vi "bumper d.vi"() -> ()   [LabVIEW 2013]
uses:
  <vilib>/NXT/Block Support/NXT_InputPort.ctl
  <vilib>/NXT/Block Support/NXT_MessageMailbox.ctl
  <vilib>/NXT/Subs/MotorOutput.ctl
  <vilib>/NXT/Block Support/NXT_OutputPort.ctl
  <vilib>/NXT/Dual Mode Library/BT/BlueTooth_Write_Num.vi
  <vilib>/NXT/Dual Mode Library/Display/drawNumber_float.vi
  <vilib>/NXT/Dual Mode Library/Display/drawNumber.vi
  <vilib>/NXT/Dual Mode Library/Sound/PlayRedPianoFile.vi
  <vilib>/NXT/NXTIO Xnodes/NXTIONodeSubVIs/NXTStopMotors.vi
  <vilib>/NXT/NXTIO Xnodes/AddressXNode/NXTIOAddress.xnode
  <vilib>/NXT/NXTIO Xnodes/NXTIOXNode/NXTIO.xnode
  <vilib>/NXT/Subs/LVHSConnector.ctl
  <vilib>/NXT/LegoClasses/BrickReference/BrickReference.lvclass
panel:
  out "Case Accord. BJr.":i32
  out "touch right":bool
  out "touch left":bool
  in  "threshold steer":dbl=0.2
  out "norm dist":dbl
  out "right dist":i16
  out "left dist":i16
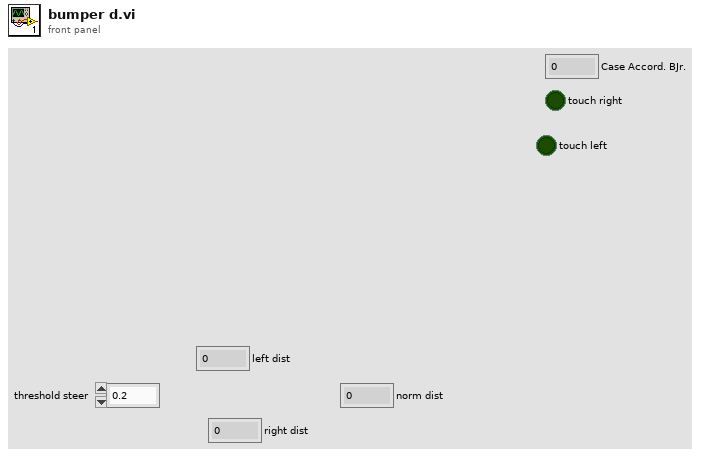
[diagram p1: front panel]
types:
  T1 = typedef "NXT_OutputPort.ctl" = u8
  T2 = typedef "NXT_MessageMailbox.ctl" = u8
  T3 = typedef "NXT_InputPort.ctl" = u32
  T4 = typedef "LVHSConnector.ctl" = refnum<class "BrickReference.lvclass">
  T5 = typedef "MotorOutput.ctl" = u8
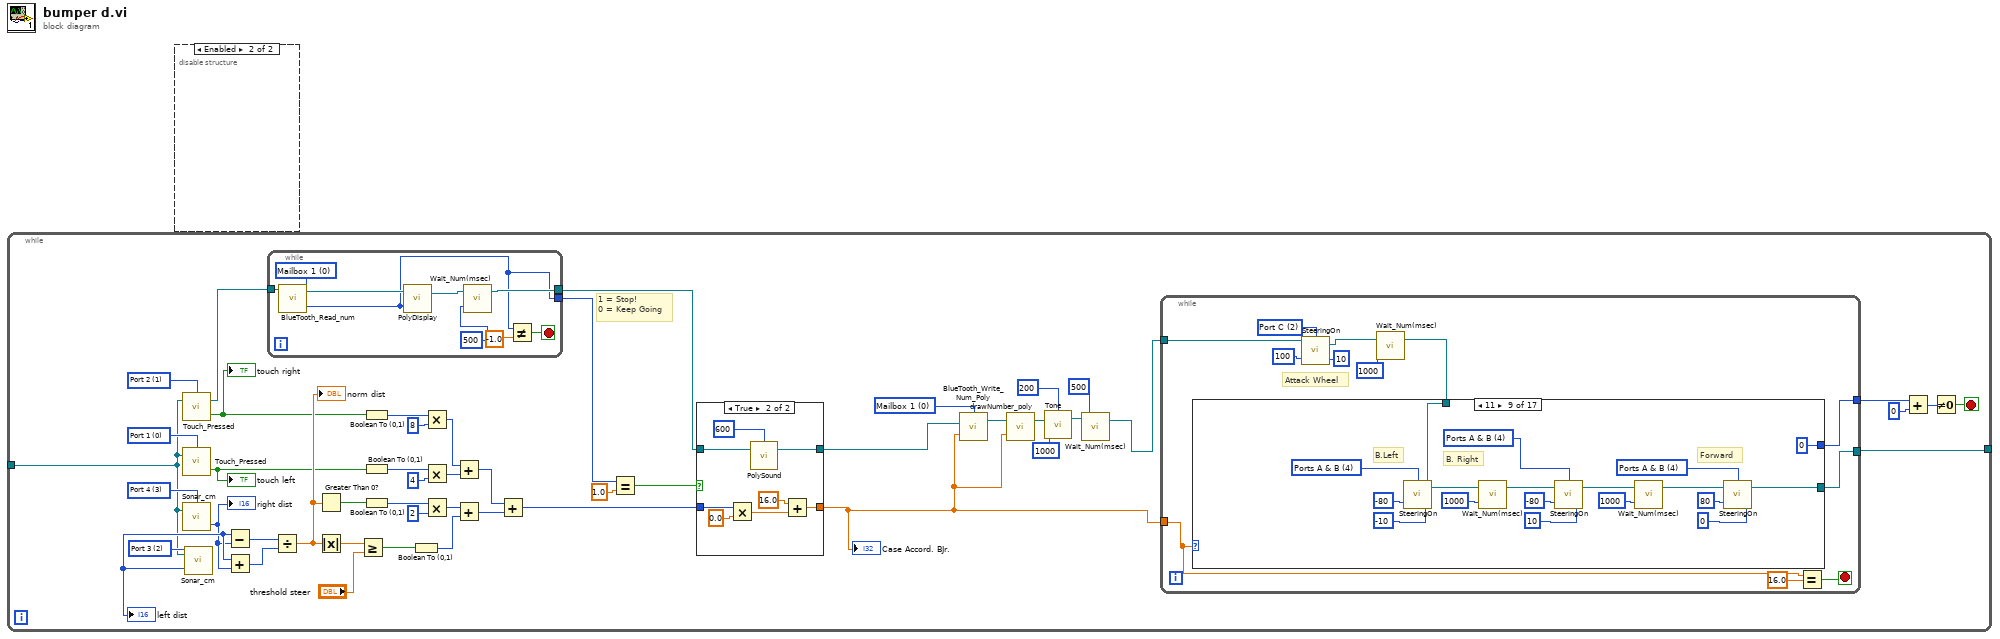
[diagram p0: block diagram]
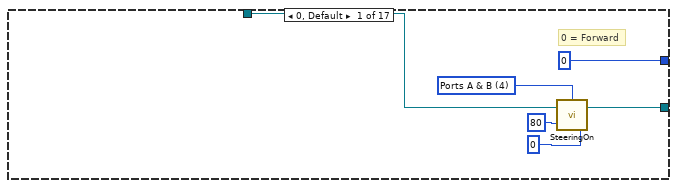
[diagram p3: hidden frame]
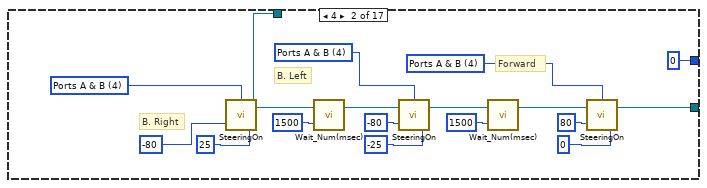
[diagram p4: hidden frame]
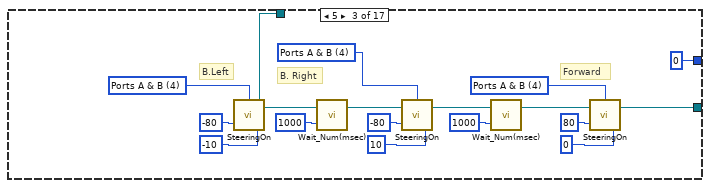
[diagram p5: hidden frame]
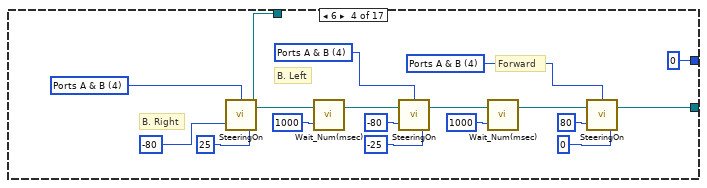
[diagram p6: hidden frame]
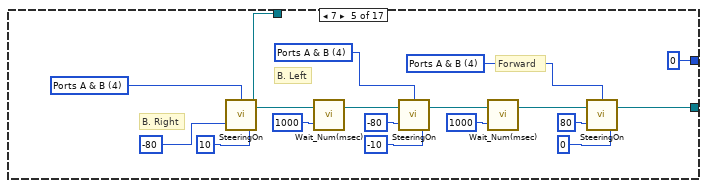
[diagram p7: hidden frame]
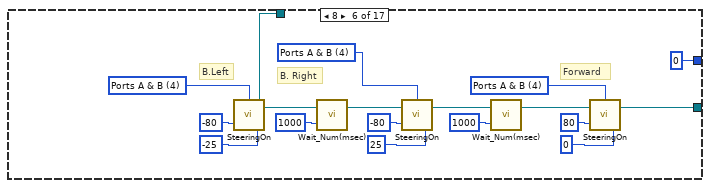
[diagram p8: hidden frame]
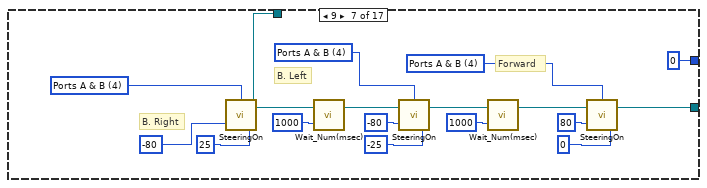
[diagram p9: hidden frame]
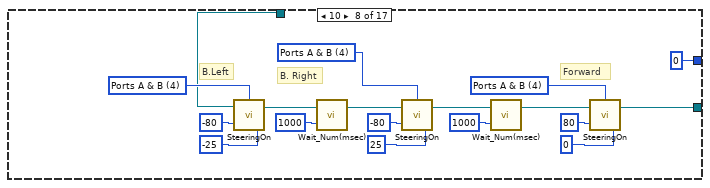
[diagram p10: hidden frame]
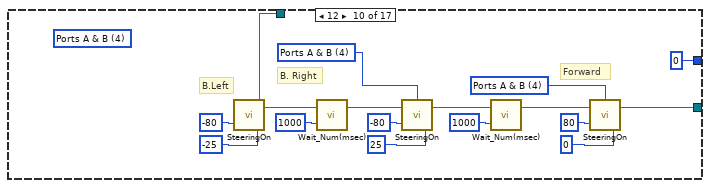
[diagram p11: hidden frame]
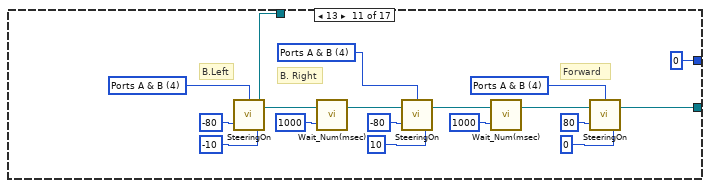
[diagram p12: hidden frame]
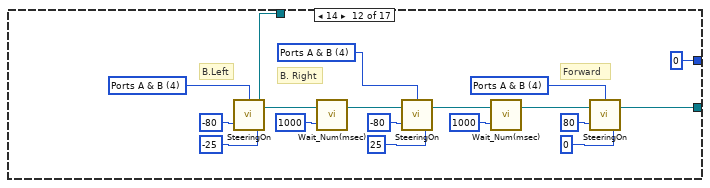
[diagram p13: hidden frame]
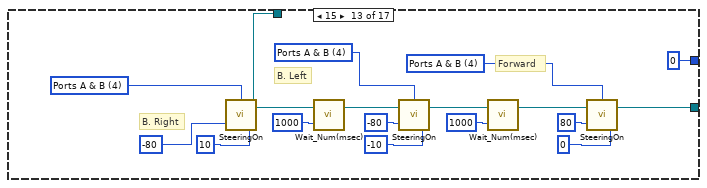
[diagram p14: hidden frame]
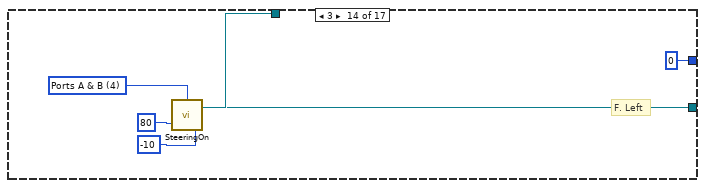
[diagram p15: hidden frame]
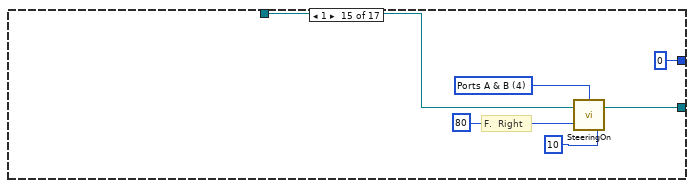
[diagram p16: hidden frame]
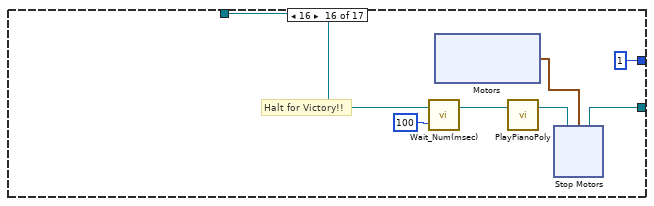
[diagram p17: hidden frame]
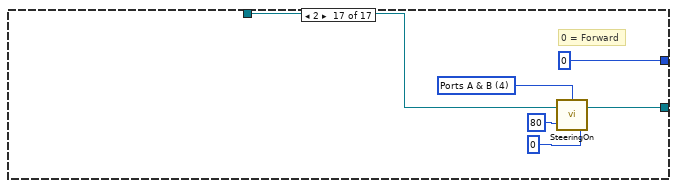
[diagram p18: hidden frame]
diagram:
  n1 = while {
    tunnel: [w15] -> _
    tunnel: [w5] -> _
    stop <- w17 stop-if-true
    w11 = T2 0 items=["Mailbox 1", "Mailbox 2", "Mailbox 3", "Mailbox 4", "Mailbox 5", "Mailbox 6", "Mailbox 7", "Mailbox 8", "Mailbox 9", "Mailbox 10"] ("Mailbox")
    w39 = T3 1 items=["Port 1", "Port 2", "Port 3", "Port 4"] ("Port (Port 1)")
    w40 = T3 0 items=["Port 1", "Port 2", "Port 3", "Port 4"] ("Port (Port 1)")
    w48 = T3 3 items=["Port 1", "Port 2", "Port 3", "Port 4"] ("Port (Port 4)")
    w49 = T3 2 items=["Port 1", "Port 2", "Port 3", "Port 4"] ("Port (Port 4)")
    # "1 = Stop!\n0 = Keep Going"
    n2 = call <vilib>:"Sonar_cm.vi"("Port (Port 4)"=w49) -> ("Distance (cm)"=w47:i16, "NXT/EV3"=w15:T4)  [unwired: 2 in]
    "left dist" <- w47
    n3 = call <vilib>:"Touch_Pressed.vi"("NXT/EV3"=w15, "Port (Port 1)"=w39) -> ("Yes / No"=w25:bool, "NXT/EV3"=w13:T4)  [unwired: 1 in]
    "touch right" <- w25
    n4 = call <vilib>:"Touch_Pressed.vi"("NXT/EV3"=w15, "Port (Port 1)"=w40) -> ("Yes / No"=w26:bool)  [unwired: 1 in, 1 out]
    "touch left" <- w26
    n5 = call <vilib>:"Sonar_cm.vi"("NXT/EV3"=w15, "Port (Port 4)"=w48) -> ("Distance (cm)"=w46:i16)  [unwired: 1 in, 1 out]
    "right dist" <- w46
    n6 = Subtract(x=w47, y=w46) -> (x-y=w45:i16)
    n7 = Add(x=w47, y=w46) -> (x+y=w44:i16)
    n8 = while {
      tunnel: w13 -> [w318]
      tunnel: [w314] -> w21
      tunnel: [w315] -> w14
      stop <- w321 stop-if-true
      w317 = T2 0 items=["Mailbox 1", "Mailbox 2", "Mailbox 3", "Mailbox 4", "Mailbox 5", "Mailbox 6", "Mailbox 7", "Mailbox 8", "Mailbox 9", "Mailbox 10"] ("Mailbox")
      n9 = call <vilib>:"BlueTooth_Read_num.vi"("NXT/EV3"=w318, "Mailbox"=w317) -> ("Message"=w314:i32, "NXT/EV3"=w320:T4)  [unwired: 1 in]
      n10 = call-poly <vilib>:"PolyDisplay.vi"("number"=w314, "NXT/EV3"=w320) -> ("NXT/EV3"=w319:T4)  [unwired: 2 in]
      n11 = call <vilib>:"Wait_Num(msec).vi"("Time (100 msec)"=u32 500, "NXT/EV3"=w319) -> ("NXT/EV3"=w315:T4)  [unwired: 2 in]
      n12 = Not Equal?(x=w314, y=-1.0) -> (x != y?=w321:bool)
    }
    n13 = Divide(x=w45, y=w44) -> (x/y=w41:dbl)
    "norm dist" <- w41
    n14 = Greater Than 0?(x=w41) -> (x > 0?=w24:bool)
    n15 = Absolute Value(x=w41) -> (abs(x)=w43:dbl)
    n16 = Greater Or Equal?(x=w43, y="threshold steer") -> (x >= y?=w23:bool)
    n17 = Boolean To (0,1)(Boolean=w25) -> (0, 1=w34:i16)
    n18 = Boolean To (0,1)(Boolean=w26) -> (0, 1=w33:i16)
    n19 = Boolean To (0,1)(Boolean=w24) -> (0, 1=w38:i16)
    n20 = Boolean To (0,1)(Boolean=w23) -> (0, 1=w28:i16)
    n21 = Multiply(x=w34, y=i16 8) -> (x*y=w31:i16)
    n22 = Multiply(x=w33, y=i16 4) -> (x*y=w30:i16)
    n23 = Multiply(x=w38, y=i16 2) -> (x*y=w29:i16)
    n24 = Add(x=w31, y=w30) -> (x+y=w32:i16)
    n25 = Add(x=w29, y=w28) -> (x+y=w27:i16)
    n26 = Add(x=w32, y=w27) -> (x+y=w16:i16)
    n27 = Equal?(x=w21, y=1.0) -> (x = y?=w20:bool)
    n28 = case shown="True" w20 {
      tunnel: w16 -> [w324 w330]
      tunnel: [w324 w325] -> w7
      tunnel: w14 -> [w323 w329]
      tunnel: [w323 w328] -> w9
      frame False {
      }
      frame True {
        n29 = Multiply(x=w330, y=0.0) -> (x*y=w327:dbl)
        n30 = call-poly <vilib>:"PolySound.vi"("NXT/EV3"=w329, "Tone (440 Hz)"=u16 600) -> ("NXT/EV3"=w328:T4)  [unwired: 2 in]
        n31 = Add(x=16.0, y=w327) -> (x+y=w325:dbl)
      }
    }
    "Case Accord. BJr." <- w7
    n32 = call-poly <vilib>:"BlueTooth_Write_Num_Poly.vi"("Message"=w7, "NXT/EV3"=w9, "Mailbox"=w11) -> ("NXT/EV3"=w12:T4)  [unwired: 1 in]
    n33 = call-poly <vilib>:"drawNumber_poly.vi"("number"=w7, "NXT/EV3"=w12) -> ("NXT/EV3"=w3:T4)  [unwired: 2 in]
    n34 = call <vilib>:"Tone.vi"("Duration (500 ms)"=u16 1000, "NXT/EV3"=w3, "Tone (440 Hz)"=u16 200) -> ("NXT/EV3"=w2:T4)  [unwired: 1 in]
    n35 = call <vilib>:"Wait_Num(msec).vi"("Time (100 msec)"=u32 500, "NXT/EV3"=w2) -> ("NXT/EV3"=w8:T4)  [unwired: 2 in]
    n36 = while {
      tunnel: w8 -> [w58]
      tunnel: w7 -> [w53]
      tunnel: [w57] -> w6
      tunnel: [w56] -> w5
      stop <- w55 stop-if-true
      w61 = T5 2 items=["Port A"=0, "Port B"=1, "Port C"=2, "Ports A & B"=4, "Ports A & C"=5, "Ports B & C"=6, "All Ports"=3] ("Output Ports (A & B)")
      # "Attack Wheel"
      n37 = call <vilib>:"SteeringOn.vi"("Power (75)"=100, "Steering (100)"=10, "NXT/EV3"=w58, "Output Ports (A & B)"=w61) -> ("NXT/EV3"=w52:T4)
      n38 = call <vilib>:"Wait_Num(msec).vi"("Time (100 msec)"=u32 1000, "NXT/EV3"=w52) -> ("NXT/EV3"=w51:T4)  [unwired: 2 in]
      n39 = case shown="11" w53 {
        tunnel: w51 -> [w65 w79 w88 w106 w124 w151 w160 w178 w196 w214 w231 w249 w268 w286 w292 w295 w311]
        tunnel: [w64 w78 w87 w105 w123 w150 w159 w177 w195 w213 w230 w248 w267 w285 w291 w298 w310] -> w56
        tunnel: [0 ("y") 0 ("y") 0 ("y") 0 ("y") 0 ("y") 0 ("y") 0 ("y") 0 ("y") 0 ("y") 0 ("y") 0 ("y") 0 ("y") 0 ("y") 0 ("y") 0 1 0 ("y")] -> w57
        frame 0, Default {
          w63 = T5 4 items=["Port A"=0, "Port B"=1, "Port C"=2, "Ports A & B"=4, "Ports A & C"=5, "Ports B & C"=6, "All Ports"=3] ("Output Ports (A & B) 5")
          # "0 = Forward"
          n40 = call <vilib>:"SteeringOn.vi"("Power (75)"=80, "Steering (100)"=0, "NXT/EV3"=w65, "Output Ports (A & B)"=w63) -> ("NXT/EV3"=w64:T4)
        }
        frame 4 {
          w75 = T5 4 items=["Port A"=0, "Port B"=1, "Port C"=2, "Ports A & B"=4, "Ports A & C"=5, "Ports B & C"=6, "All Ports"=3] ("Output Ports (A & B) 15")
          w76 = T5 4 items=["Port A"=0, "Port B"=1, "Port C"=2, "Ports A & B"=4, "Ports A & C"=5, "Ports B & C"=6, "All Ports"=3] ("Output Port (All Ports) 6")
          w77 = T5 4 items=["Port A"=0, "Port B"=1, "Port C"=2, "Ports A & B"=4, "Ports A & C"=5, "Ports B & C"=6, "All Ports"=3] ("Output Ports (A & B) 16")
          # "Forward"
          # "B. Left"
          # "B. Right"
          n41 = call <vilib>:"SteeringOn.vi"("Power (75)"=-80, "Steering (100)"=25, "NXT/EV3"=w79, "Output Ports (A & B)"=w77) -> ("NXT/EV3"=w74:T4)
          n42 = call <vilib>:"Wait_Num(msec).vi"("Time (100 msec)"=u32 1500, "NXT/EV3"=w74) -> ("NXT/EV3"=w73:T4)  [unwired: 2 in]
          n43 = call <vilib>:"SteeringOn.vi"("Power (75)"=-80, "Steering (100)"=-25, "NXT/EV3"=w73, "Output Ports (A & B)"=w76) -> ("NXT/EV3"=w72:T4)
          n44 = call <vilib>:"Wait_Num(msec).vi"("Time (100 msec)"=u32 1500, "NXT/EV3"=w72) -> ("NXT/EV3"=w71:T4)  [unwired: 2 in]
          n45 = call <vilib>:"SteeringOn.vi"("Power (75)"=80, "Steering (100)"=0, "NXT/EV3"=w71, "Output Ports (A & B)"=w75) -> ("NXT/EV3"=w78:T4)
        }
        frame 5 {
          w95 = T5 4 items=["Port A"=0, "Port B"=1, "Port C"=2, "Ports A & B"=4, "Ports A & C"=5, "Ports B & C"=6, "All Ports"=3] ("Output Ports (A & B) 21")
          w96 = T5 4 items=["Port A"=0, "Port B"=1, "Port C"=2, "Ports A & B"=4, "Ports A & C"=5, "Ports B & C"=6, "All Ports"=3] ("Output Port (All Ports) 9")
          w97 = T5 4 items=["Port A"=0, "Port B"=1, "Port C"=2, "Ports A & B"=4, "Ports A & C"=5, "Ports B & C"=6, "All Ports"=3] ("Output Ports (A & B) 22")
          # "Forward"
          # "B. Right"
          # "B.Left"
          n46 = call <vilib>:"SteeringOn.vi"("Power (75)"=-80, "Steering (100)"=-10, "NXT/EV3"=w88, "Output Ports (A & B)"=w97) -> ("NXT/EV3"=w93:T4)
          n47 = call <vilib>:"Wait_Num(msec).vi"("Time (100 msec)"=u32 1000, "NXT/EV3"=w93) -> ("NXT/EV3"=w92:T4)  [unwired: 2 in]
          n48 = call <vilib>:"SteeringOn.vi"("Power (75)"=-80, "Steering (100)"=10, "NXT/EV3"=w92, "Output Ports (A & B)"=w96) -> ("NXT/EV3"=w90:T4)
          n49 = call <vilib>:"Wait_Num(msec).vi"("Time (100 msec)"=u32 1000, "NXT/EV3"=w90) -> ("NXT/EV3"=w89:T4)  [unwired: 2 in]
          n50 = call <vilib>:"SteeringOn.vi"("Power (75)"=80, "Steering (100)"=0, "NXT/EV3"=w89, "Output Ports (A & B)"=w95) -> ("NXT/EV3"=w87:T4)
        }
        frame 6 {
          w115 = T5 4 items=["Port A"=0, "Port B"=1, "Port C"=2, "Ports A & B"=4, "Ports A & C"=5, "Ports B & C"=6, "All Ports"=3] ("Output Ports (A & B) 15")
          w114 = T5 4 items=["Port A"=0, "Port B"=1, "Port C"=2, "Ports A & B"=4, "Ports A & C"=5, "Ports B & C"=6, "All Ports"=3] ("Output Port (All Ports) 6")
          w113 = T5 4 items=["Port A"=0, "Port B"=1, "Port C"=2, "Ports A & B"=4, "Ports A & C"=5, "Ports B & C"=6, "All Ports"=3] ("Output Ports (A & B) 16")
          # "Forward"
          # "B. Left"
          # "B. Right"
          n51 = call <vilib>:"SteeringOn.vi"("Power (75)"=-80, "Steering (100)"=25, "NXT/EV3"=w106, "Output Ports (A & B)"=w113) -> ("NXT/EV3"=w116:T4)
          n52 = call <vilib>:"Wait_Num(msec).vi"("Time (100 msec)"=u32 1000, "NXT/EV3"=w116) -> ("NXT/EV3"=w117:T4)  [unwired: 2 in]
          n53 = call <vilib>:"SteeringOn.vi"("Power (75)"=-80, "Steering (100)"=-25, "NXT/EV3"=w117, "Output Ports (A & B)"=w114) -> ("NXT/EV3"=w118:T4)
          n54 = call <vilib>:"Wait_Num(msec).vi"("Time (100 msec)"=u32 1000, "NXT/EV3"=w118) -> ("NXT/EV3"=w119:T4)  [unwired: 2 in]
          n55 = call <vilib>:"SteeringOn.vi"("Power (75)"=80, "Steering (100)"=0, "NXT/EV3"=w119, "Output Ports (A & B)"=w115) -> ("NXT/EV3"=w105:T4)
        }
        frame 7 {
          w133 = T5 4 items=["Port A"=0, "Port B"=1, "Port C"=2, "Ports A & B"=4, "Ports A & C"=5, "Ports B & C"=6, "All Ports"=3] ("Output Ports (A & B) 15")
          w132 = T5 4 items=["Port A"=0, "Port B"=1, "Port C"=2, "Ports A & B"=4, "Ports A & C"=5, "Ports B & C"=6, "All Ports"=3] ("Output Port (All Ports) 6")
          w131 = T5 4 items=["Port A"=0, "Port B"=1, "Port C"=2, "Ports A & B"=4, "Ports A & C"=5, "Ports B & C"=6, "All Ports"=3] ("Output Ports (A & B) 16")
          # "Forward"
          # "B. Left"
          # "B. Right"
          n56 = call <vilib>:"SteeringOn.vi"("Power (75)"=-80, "Steering (100)"=10, "NXT/EV3"=w124, "Output Ports (A & B)"=w131) -> ("NXT/EV3"=w134:T4)
          n57 = call <vilib>:"Wait_Num(msec).vi"("Time (100 msec)"=u32 1000, "NXT/EV3"=w134) -> ("NXT/EV3"=w135:T4)  [unwired: 2 in]
          n58 = call <vilib>:"SteeringOn.vi"("Power (75)"=-80, "Steering (100)"=-10, "NXT/EV3"=w135, "Output Ports (A & B)"=w132) -> ("NXT/EV3"=w136:T4)
          n59 = call <vilib>:"Wait_Num(msec).vi"("Time (100 msec)"=u32 1000, "NXT/EV3"=w136) -> ("NXT/EV3"=w137:T4)  [unwired: 2 in]
          n60 = call <vilib>:"SteeringOn.vi"("Power (75)"=80, "Steering (100)"=0, "NXT/EV3"=w137, "Output Ports (A & B)"=w133) -> ("NXT/EV3"=w123:T4)
        }
        frame 8 {
          w147 = T5 4 items=["Port A"=0, "Port B"=1, "Port C"=2, "Ports A & B"=4, "Ports A & C"=5, "Ports B & C"=6, "All Ports"=3] ("Output Ports (A & B) 21")
          w148 = T5 4 items=["Port A"=0, "Port B"=1, "Port C"=2, "Ports A & B"=4, "Ports A & C"=5, "Ports B & C"=6, "All Ports"=3] ("Output Port (All Ports) 9")
          w149 = T5 4 items=["Port A"=0, "Port B"=1, "Port C"=2, "Ports A & B"=4, "Ports A & C"=5, "Ports B & C"=6, "All Ports"=3] ("Output Ports (A & B) 22")
          # "Forward"
          # "B. Right"
          # "B.Left"
          n61 = call <vilib>:"SteeringOn.vi"("Power (75)"=-80, "Steering (100)"=-25, "NXT/EV3"=w151, "Output Ports (A & B)"=w149) -> ("NXT/EV3"=w145:T4)
          n62 = call <vilib>:"Wait_Num(msec).vi"("Time (100 msec)"=u32 1000, "NXT/EV3"=w145) -> ("NXT/EV3"=w144:T4)  [unwired: 2 in]
          n63 = call <vilib>:"SteeringOn.vi"("Power (75)"=-80, "Steering (100)"=25, "NXT/EV3"=w144, "Output Ports (A & B)"=w148) -> ("NXT/EV3"=w142:T4)
          n64 = call <vilib>:"Wait_Num(msec).vi"("Time (100 msec)"=u32 1000, "NXT/EV3"=w142) -> ("NXT/EV3"=w141:T4)  [unwired: 2 in]
          n65 = call <vilib>:"SteeringOn.vi"("Power (75)"=80, "Steering (100)"=0, "NXT/EV3"=w141, "Output Ports (A & B)"=w147) -> ("NXT/EV3"=w150:T4)
        }
        frame 9 {
          w167 = T5 4 items=["Port A"=0, "Port B"=1, "Port C"=2, "Ports A & B"=4, "Ports A & C"=5, "Ports B & C"=6, "All Ports"=3] ("Output Ports (A & B) 15")
          w168 = T5 4 items=["Port A"=0, "Port B"=1, "Port C"=2, "Ports A & B"=4, "Ports A & C"=5, "Ports B & C"=6, "All Ports"=3] ("Output Port (All Ports) 6")
          w169 = T5 4 items=["Port A"=0, "Port B"=1, "Port C"=2, "Ports A & B"=4, "Ports A & C"=5, "Ports B & C"=6, "All Ports"=3] ("Output Ports (A & B) 16")
          # "Forward"
          # "B. Left"
          # "B. Right"
          n66 = call <vilib>:"SteeringOn.vi"("Power (75)"=-80, "Steering (100)"=25, "NXT/EV3"=w160, "Output Ports (A & B)"=w169) -> ("NXT/EV3"=w166:T4)
          n67 = call <vilib>:"Wait_Num(msec).vi"("Time (100 msec)"=u32 1000, "NXT/EV3"=w166) -> ("NXT/EV3"=w165:T4)  [unwired: 2 in]
          n68 = call <vilib>:"SteeringOn.vi"("Power (75)"=-80, "Steering (100)"=-25, "NXT/EV3"=w165, "Output Ports (A & B)"=w168) -> ("NXT/EV3"=w164:T4)
          n69 = call <vilib>:"Wait_Num(msec).vi"("Time (100 msec)"=u32 1000, "NXT/EV3"=w164) -> ("NXT/EV3"=w163:T4)  [unwired: 2 in]
          n70 = call <vilib>:"SteeringOn.vi"("Power (75)"=80, "Steering (100)"=0, "NXT/EV3"=w163, "Output Ports (A & B)"=w167) -> ("NXT/EV3"=w159:T4)
        }
        frame 10 {
          w187 = T5 4 items=["Port A"=0, "Port B"=1, "Port C"=2, "Ports A & B"=4, "Ports A & C"=5, "Ports B & C"=6, "All Ports"=3] ("Output Ports (A & B) 21")
          w186 = T5 4 items=["Port A"=0, "Port B"=1, "Port C"=2, "Ports A & B"=4, "Ports A & C"=5, "Ports B & C"=6, "All Ports"=3] ("Output Port (All Ports) 9")
          w185 = T5 4 items=["Port A"=0, "Port B"=1, "Port C"=2, "Ports A & B"=4, "Ports A & C"=5, "Ports B & C"=6, "All Ports"=3] ("Output Ports (A & B) 22")
          # "Forward"
          # "B. Right"
          # "B.Left"
          n71 = call <vilib>:"SteeringOn.vi"("Power (75)"=-80, "Steering (100)"=-25, "NXT/EV3"=w178, "Output Ports (A & B)"=w185) -> ("NXT/EV3"=w189:T4)
          n72 = call <vilib>:"Wait_Num(msec).vi"("Time (100 msec)"=u32 1000, "NXT/EV3"=w189) -> ("NXT/EV3"=w190:T4)  [unwired: 2 in]
          n73 = call <vilib>:"SteeringOn.vi"("Power (75)"=-80, "Steering (100)"=25, "NXT/EV3"=w190, "Output Ports (A & B)"=w186) -> ("NXT/EV3"=w192:T4)
          n74 = call <vilib>:"Wait_Num(msec).vi"("Time (100 msec)"=u32 1000, "NXT/EV3"=w192) -> ("NXT/EV3"=w193:T4)  [unwired: 2 in]
          n75 = call <vilib>:"SteeringOn.vi"("Power (75)"=80, "Steering (100)"=0, "NXT/EV3"=w193, "Output Ports (A & B)"=w187) -> ("NXT/EV3"=w177:T4)
        }
        frame 11 {
          w205 = T5 4 items=["Port A"=0, "Port B"=1, "Port C"=2, "Ports A & B"=4, "Ports A & C"=5, "Ports B & C"=6, "All Ports"=3] ("Output Ports (A & B) 21")
          w204 = T5 4 items=["Port A"=0, "Port B"=1, "Port C"=2, "Ports A & B"=4, "Ports A & C"=5, "Ports B & C"=6, "All Ports"=3] ("Output Port (All Ports) 9")
          w203 = T5 4 items=["Port A"=0, "Port B"=1, "Port C"=2, "Ports A & B"=4, "Ports A & C"=5, "Ports B & C"=6, "All Ports"=3] ("Output Ports (A & B) 22")
          # "Forward"
          # "B. Right"
          # "B.Left"
          n76 = call <vilib>:"SteeringOn.vi"("Power (75)"=-80, "Steering (100)"=-10, "NXT/EV3"=w196, "Output Ports (A & B)"=w203) -> ("NXT/EV3"=w207:T4)
          n77 = call <vilib>:"Wait_Num(msec).vi"("Time (100 msec)"=u32 1000, "NXT/EV3"=w207) -> ("NXT/EV3"=w208:T4)  [unwired: 2 in]
          n78 = call <vilib>:"SteeringOn.vi"("Power (75)"=-80, "Steering (100)"=10, "NXT/EV3"=w208, "Output Ports (A & B)"=w204) -> ("NXT/EV3"=w210:T4)
          n79 = call <vilib>:"Wait_Num(msec).vi"("Time (100 msec)"=u32 1000, "NXT/EV3"=w210) -> ("NXT/EV3"=w211:T4)  [unwired: 2 in]
          n80 = call <vilib>:"SteeringOn.vi"("Power (75)"=80, "Steering (100)"=0, "NXT/EV3"=w211, "Output Ports (A & B)"=w205) -> ("NXT/EV3"=w195:T4)
        }
        frame 12 {
          w222 = T5 4 items=["Port A"=0, "Port B"=1, "Port C"=2, "Ports A & B"=4, "Ports A & C"=5, "Ports B & C"=6, "All Ports"=3] ("Output Ports (A & B) 21")
          w221 = T5 4 items=["Port A"=0, "Port B"=1, "Port C"=2, "Ports A & B"=4, "Ports A & C"=5, "Ports B & C"=6, "All Ports"=3] ("Output Port (All Ports) 9")
          (unwired) T5 4 items=["Port A"=0, "Port B"=1, "Port C"=2, "Ports A & B"=4, "Ports A & C"=5, "Ports B & C"=6, "All Ports"=3] ("Output Ports (A & B) 22")
          # "Forward"
          # "B. Right"
          # "B.Left"
          n81 = call <vilib>:"SteeringOn.vi"("Power (75)"=-80, "Steering (100)"=-25, "NXT/EV3"=w214) -> ("NXT/EV3"=w224:T4)  [unwired: 1 in]
          n82 = call <vilib>:"Wait_Num(msec).vi"("Time (100 msec)"=u32 1000, "NXT/EV3"=w224) -> ("NXT/EV3"=w225:T4)  [unwired: 2 in]
          n83 = call <vilib>:"SteeringOn.vi"("Power (75)"=-80, "Steering (100)"=25, "NXT/EV3"=w225, "Output Ports (A & B)"=w221) -> ("NXT/EV3"=w227:T4)
          n84 = call <vilib>:"Wait_Num(msec).vi"("Time (100 msec)"=u32 1000, "NXT/EV3"=w227) -> ("NXT/EV3"=w228:T4)  [unwired: 2 in]
          n85 = call <vilib>:"SteeringOn.vi"("Power (75)"=80, "Steering (100)"=0, "NXT/EV3"=w228, "Output Ports (A & B)"=w222) -> ("NXT/EV3"=w213:T4)
        }
        frame 13 {
          w238 = T5 4 items=["Port A"=0, "Port B"=1, "Port C"=2, "Ports A & B"=4, "Ports A & C"=5, "Ports B & C"=6, "All Ports"=3] ("Output Ports (A & B) 21")
          w239 = T5 4 items=["Port A"=0, "Port B"=1, "Port C"=2, "Ports A & B"=4, "Ports A & C"=5, "Ports B & C"=6, "All Ports"=3] ("Output Port (All Ports) 9")
          w240 = T5 4 items=["Port A"=0, "Port B"=1, "Port C"=2, "Ports A & B"=4, "Ports A & C"=5, "Ports B & C"=6, "All Ports"=3] ("Output Ports (A & B) 22")
          # "Forward"
          # "B. Right"
          # "B.Left"
          n86 = call <vilib>:"SteeringOn.vi"("Power (75)"=-80, "Steering (100)"=-10, "NXT/EV3"=w231, "Output Ports (A & B)"=w240) -> ("NXT/EV3"=w236:T4)
          n87 = call <vilib>:"Wait_Num(msec).vi"("Time (100 msec)"=u32 1000, "NXT/EV3"=w236) -> ("NXT/EV3"=w235:T4)  [unwired: 2 in]
          n88 = call <vilib>:"SteeringOn.vi"("Power (75)"=-80, "Steering (100)"=10, "NXT/EV3"=w235, "Output Ports (A & B)"=w239) -> ("NXT/EV3"=w233:T4)
          n89 = call <vilib>:"Wait_Num(msec).vi"("Time (100 msec)"=u32 1000, "NXT/EV3"=w233) -> ("NXT/EV3"=w232:T4)  [unwired: 2 in]
          n90 = call <vilib>:"SteeringOn.vi"("Power (75)"=80, "Steering (100)"=0, "NXT/EV3"=w232, "Output Ports (A & B)"=w238) -> ("NXT/EV3"=w230:T4)
        }
        frame 14 {
          w258 = T5 4 items=["Port A"=0, "Port B"=1, "Port C"=2, "Ports A & B"=4, "Ports A & C"=5, "Ports B & C"=6, "All Ports"=3] ("Output Ports (A & B) 21")
          w257 = T5 4 items=["Port A"=0, "Port B"=1, "Port C"=2, "Ports A & B"=4, "Ports A & C"=5, "Ports B & C"=6, "All Ports"=3] ("Output Port (All Ports) 9")
          w256 = T5 4 items=["Port A"=0, "Port B"=1, "Port C"=2, "Ports A & B"=4, "Ports A & C"=5, "Ports B & C"=6, "All Ports"=3] ("Output Ports (A & B) 22")
          # "Forward"
          # "B. Right"
          # "B.Left"
          n91 = call <vilib>:"SteeringOn.vi"("Power (75)"=-80, "Steering (100)"=-25, "NXT/EV3"=w249, "Output Ports (A & B)"=w256) -> ("NXT/EV3"=w260:T4)
          n92 = call <vilib>:"Wait_Num(msec).vi"("Time (100 msec)"=u32 1000, "NXT/EV3"=w260) -> ("NXT/EV3"=w261:T4)  [unwired: 2 in]
          n93 = call <vilib>:"SteeringOn.vi"("Power (75)"=-80, "Steering (100)"=25, "NXT/EV3"=w261, "Output Ports (A & B)"=w257) -> ("NXT/EV3"=w263:T4)
          n94 = call <vilib>:"Wait_Num(msec).vi"("Time (100 msec)"=u32 1000, "NXT/EV3"=w263) -> ("NXT/EV3"=w264:T4)  [unwired: 2 in]
          n95 = call <vilib>:"SteeringOn.vi"("Power (75)"=80, "Steering (100)"=0, "NXT/EV3"=w264, "Output Ports (A & B)"=w258) -> ("NXT/EV3"=w248:T4)
        }
        frame 15 {
          w275 = T5 4 items=["Port A"=0, "Port B"=1, "Port C"=2, "Ports A & B"=4, "Ports A & C"=5, "Ports B & C"=6, "All Ports"=3] ("Output Ports (A & B) 15")
          w276 = T5 4 items=["Port A"=0, "Port B"=1, "Port C"=2, "Ports A & B"=4, "Ports A & C"=5, "Ports B & C"=6, "All Ports"=3] ("Output Port (All Ports) 6")
          w266 = T5 4 items=["Port A"=0, "Port B"=1, "Port C"=2, "Ports A & B"=4, "Ports A & C"=5, "Ports B & C"=6, "All Ports"=3] ("Output Ports (A & B) 16")
          # "Forward"
          # "B. Left"
          # "B. Right"
          n96 = call <vilib>:"SteeringOn.vi"("Power (75)"=-80, "Steering (100)"=10, "NXT/EV3"=w268, "Output Ports (A & B)"=w266) -> ("NXT/EV3"=w274:T4)
          n97 = call <vilib>:"Wait_Num(msec).vi"("Time (100 msec)"=u32 1000, "NXT/EV3"=w274) -> ("NXT/EV3"=w273:T4)  [unwired: 2 in]
          n98 = call <vilib>:"SteeringOn.vi"("Power (75)"=-80, "Steering (100)"=-10, "NXT/EV3"=w273, "Output Ports (A & B)"=w276) -> ("NXT/EV3"=w272:T4)
          n99 = call <vilib>:"Wait_Num(msec).vi"("Time (100 msec)"=u32 1000, "NXT/EV3"=w272) -> ("NXT/EV3"=w271:T4)  [unwired: 2 in]
          n100 = call <vilib>:"SteeringOn.vi"("Power (75)"=80, "Steering (100)"=0, "NXT/EV3"=w271, "Output Ports (A & B)"=w275) -> ("NXT/EV3"=w267:T4)
        }
        frame 3 {
          w284 = T5 4 items=["Port A"=0, "Port B"=1, "Port C"=2, "Ports A & B"=4, "Ports A & C"=5, "Ports B & C"=6, "All Ports"=3] ("Output Port (All Ports) 3")
          # "F. Left"
          n101 = call <vilib>:"SteeringOn.vi"("Power (75)"=80, "Steering (100)"=-10, "NXT/EV3"=w286, "Output Ports (A & B)"=w284) -> ("NXT/EV3"=w285:T4)
        }
        frame 1 {
          w290 = T5 4 items=["Port A"=0, "Port B"=1, "Port C"=2, "Ports A & B"=4, "Ports A & C"=5, "Ports B & C"=6, "All Ports"=3] ("Output Ports (A & B) 12")
          # "F.  Right"
          n102 = call <vilib>:"SteeringOn.vi"("Power (75)"=80, "Steering (100)"=10, "NXT/EV3"=w292, "Output Ports (A & B)"=w290) -> ("NXT/EV3"=w291:T4)
        }
        frame 16 {
          # "Halt for Victory!!"
          n103 = call <vilib>:"Wait_Num(msec).vi"("Time (100 msec)"=u32 100, "NXT/EV3"=w295) -> ("NXT/EV3"=w297:T4)  [unwired: 2 in]
          n104 = xnode "Motors"() -> ("Motor"=w301:cluster{"Port":T1, "Port":T1})
          n105 = call-poly <vilib>:"PlayPianoPoly.vi"("NXT/EV3"=w297) -> ("NXT/EV3"=w296:T4)  [unwired: 3 in]
          n106 = xnode "Stop Motors"("Motors"=w301, "NXT/EV3"=w296) -> ("NXT/EV3"=w298:T4)
        }
        frame 2 {
          w309 = T5 4 items=["Port A"=0, "Port B"=1, "Port C"=2, "Ports A & B"=4, "Ports A & C"=5, "Ports B & C"=6, "All Ports"=3] ("Output Ports (A & B) 10")
          # "0 = Forward"
          n107 = call <vilib>:"SteeringOn.vi"("Power (75)"=80, "Steering (100)"=0, "NXT/EV3"=w311, "Output Ports (A & B)"=w309) -> ("NXT/EV3"=w310:T4)
        }
      }
      n108 = Equal?(x=w53, y=16.0) -> (x = y?=w55:bool)
    }
    n109 = Add(x=w6, y=0) -> (x+y=w18:i32)
    n110 = Not Equal To 0?(x=w18) -> (x != 0?=w17:bool)
  }
  n111 = disable-structure shown="Enabled" {
    frame Disabled {
    }
    frame Enabled {
    }
  }
